vi "DAQmx电压采集.vi"(7 "被测通道":tag="Dev1/ai0", 8 "error in":errorcluster caption="错误输入", 10 "设置":string[](array[string])=["160", "10", "0.02", "0.02", "0.1", "10", "J5", "J6"], 11 "参考通道":tag="Dev1/ai0") -> (0 "error out":errorcluster caption="错误输出", 1 "被测幅值":dbl format="%.2p", 2 "参考幅值":dbl format="%.2p", 4 "满足条件":bool)   [LabVIEW 2015]
uses:
  <vilib>/Utility/error.llb/DialogType.ctl
  <vilib>/DAQmx/read.llb/DAQmx Read (Analog 1D Wfm NChan NSamp).vi
  <vilib>/DAQmx/create/channels.llb/DAQmx Create Channel (AI-Voltage-Basic).vi
  <vilib>/DAQmx/create/channels.llb/DAQmx Create Channel (AI-Acceleration-Accelerometer).vi
  <vilib>/DAQmx/configure/timing.llb/DAQmx Timing (Sample Clock).vi
  <vilib>/DAQmx/miscellaneous.llb/DAQmx Fill In Error Info.vi
  <vilib>/measure/matone.llb/Extract Single Tone Information N Chan.vi
  <resource>/objmgr/daqmx.rc
  <vilib>/measure/NI_MAPro.lvlib
panel:
  out "实际采样率":dbl=1000.0 format="%0.2f"
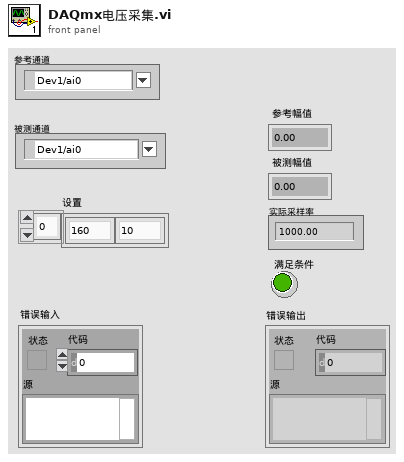
[diagram p1: front panel]
types:
  T1 = typedef "DialogType.ctl" = u16
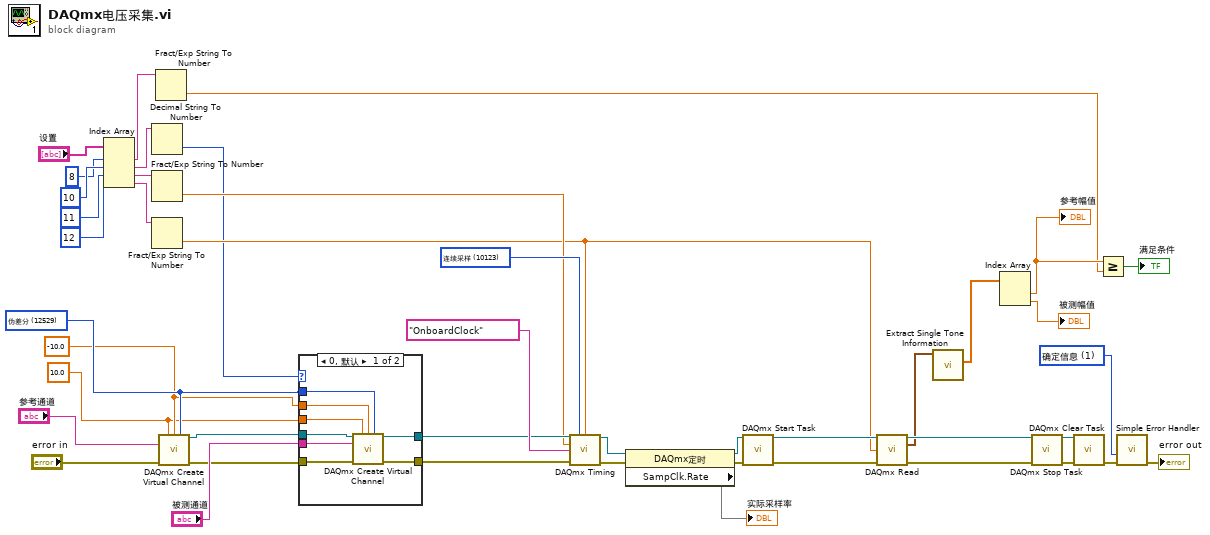
[diagram p0: block diagram]
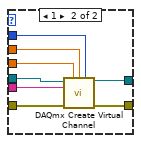
[diagram p2: hidden frame]
diagram:
  w33 = T1 1 items=["无对话框", "确定信息", "继续或停止信息", "确定信息＋警告", "继续/停止+警告"] ("type of dialog (OK msg:1)")
  w26 = 12529 items=["默认"=-1, "RSE"=10083, "NRSE"=10078, "差分"=10106, "伪差分"=12529] ("接线端配置")
  w24 = 10.0 ("最大电压")
  w25 = -10.0 ("最小电压")
  w44 = 10123 items=["有限采样"=10178, "连续采样"=10123, "硬件定时单点"=12522] ("sample mode")
  n1 = Index Array(array="设置", index #1=8 ("索引 (行)"), index #2=10 ("索引 (行)"), index #3=11 ("索引"), index #4=12 ("索引")) -> (element #1=w5:string, element #2=w15:string, element #3=w12:string, element #4=w9:string)
  n2 = Decimal String To Number(string=w15) -> (number=w4:i32)  [unwired: 2 in, 1 out]
  n3 = Fract/Exp String To Number(string=w12) -> (number=w8:dbl)  [unwired: 3 in, 1 out]
  n4 = Fract/Exp String To Number(string=w9) -> (number=w7:dbl)  [unwired: 3 in, 1 out]
  n5 = Fract/Exp String To Number(string=w5) -> (number=w2:dbl)  [unwired: 3 in, 1 out]
  n6 = call-poly <vilib>:"DAQmx Create Virtual Channel.vi"("maximum value"=w24, "minimum value"=w25, "input terminal configuration"=w26, "physical channels"="参考通道", "error in"="error in") -> ("task out"=w20:refnum<k21>, "error out"=w22:errorcluster)  [unwired: 9 in]
  n7 = case shown="0, 默认" w4 {
    tunnel: w26 -> [w52 w54]
    tunnel: w25 -> [w51 w55]
    tunnel: w24 -> [w50 w56]
    tunnel: w22 -> [w49 w59]
    tunnel: [w48 w57] -> w21
    tunnel: [w47 w58] -> w19
    tunnel: "被测通道" -> [w46 w60]
    tunnel: w20 -> [w45 w53]
    frame 0, Default {
      n8 = call-poly <vilib>:"DAQmx Create Virtual Channel.vi"("task in"=w45, "maximum value"=w50, "minimum value"=w51, "input terminal configuration"=w52, "physical channels"=w46, "error in"=w49) -> ("task out"=w47:refnum<k21>, "error out"=w48:errorcluster)  [unwired: 8 in]
    }
    frame 1 {
      n9 = call-poly <vilib>:"DAQmx Create Virtual Channel.vi"("task in"=w53, "maximum value"=w56, "minimum value"=w55, "input terminal configuration"=w54, "physical channels"=w60, "error in"=w59) -> ("task out"=w58:refnum<k21>, "error out"=w57:errorcluster)  [unwired: 8 in]
    }
  }
  n10 = call-poly <vilib>:"DAQmx Timing.vi"("task/channels in"=w19, "sample mode"=w44, "samples per channel"=w7, "rate"=w8, "source"=tag "OnboardClock" ("采样时钟源"), "error in"=w21) -> ("task out"=w35:refnum<k21>, "error out"=w38:errorcluster)  [unwired: 8 in]
  n11 = property class="DAQmx定时"(reference=w35, error in=w38) -> (reference out=w39:refnum<k21>, error out=w37:errorcluster, "SampClk.Rate"=→"实际采样率")
  n12 = call <vilib>:"DAQmx Start Task.vi"("task/channels in"=w39, "error in"=w37) -> ("task out"=w27:refnum<k21>, "error out"=w28:errorcluster)  [unwired: 12 in]
  n13 = call-poly <vilib>:"DAQmx Read.vi"("task/channels in"=w27, "number of samples per channel"=w7, "error in"=w28) -> ("task out"=w32:refnum<k21>, "data"=w18:waveform(dbl)[], "error out"=w29:errorcluster)  [unwired: 10 in]
  n14 = call-poly <vilib>:"Extract Single Tone Information.vi"("time signals in"=w18) -> ("detected amplitudes"=w17:dbl[])  [unwired: 5 in, 5 out]
  n15 = Index Array(array=w17) -> (element #1=w3:dbl, element #2=→"被测幅值":dbl)  [unwired: 2 in]
  "参考幅值" <- w3
  n16 = call <vilib>:"DAQmx Stop Task.vi"("task/channels in"=w32, "error in"=w29) -> ("task out"=w31:refnum<k21>, "error out"=w30:errorcluster)  [unwired: 12 in]
  n17 = call <vilib>:"DAQmx Clear Task.vi"("task in"=w31, "error in"=w30) -> ("error out"=w34:errorcluster)  [unwired: 13 in]
  n18 = Greater Or Equal?(x=w3, y=w2) -> (x >= y?=→"满足条件":bool)
  n19 = call <vilib>:"Simple Error Handler.vi"("type of dialog (OK msg:1)"=w33, "error in (no error)"=w34) -> ("error out"=→"error out":errorcluster)  [unwired: 3 in, 4 out]
